vi "Project - Description.vi"(7 "Msg Chain":string, 8 "error in (no error)":errorcluster {"code" format="Error %.0f"}, 10 "Project Doc":refnum<class "Project Documentation.lvclass">, 11 "VIDoc Printer - Confluence In":refnum<class "VIDoc Printer - Confluence.lvclass">) -> (0 "error out":errorcluster {"code" format="Error %.0f"}, 3 "VIDoc Printer - Confluence Out":refnum<class "VIDoc Printer - Confluence.lvclass">)   [LabVIEW 2023, in "VIDoc Printer - Confluence.lvlib" / "VIDoc Printer - Confluence.lvclass"]
uses:
  VIDoc Printer - Confluence.lvclass
  Parsing/Project Documentation/Project Documentation.lvclass
  Confluence Formatting/Types/Format Combo Box.ctl
  Parsing/Project Documentation/Project Documentation.lvclass/Project Documentation.ctl
  Parsing/Project Documentation/Get Description.vi
  VIDoc Printer - Confluence.lvclass/VIDoc Printer - Confluence.ctl
  Confluence Formatting/Confluence Formatting.lvlib
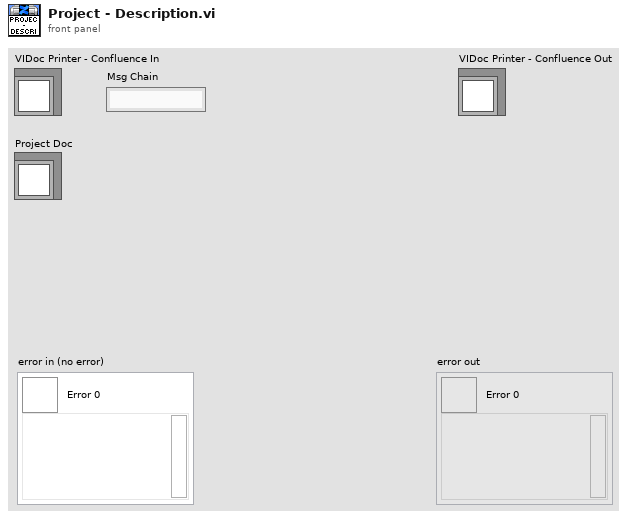
[diagram p1: front panel]
types:
  T1 = typedef "Confluence Formatting.lvlib/Format Combo Box.ctl" = string
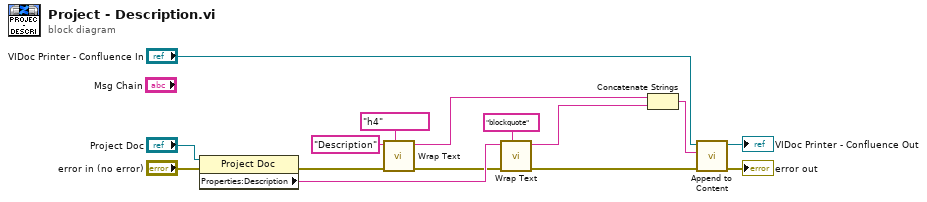
[diagram p0: block diagram]
diagram:
  n1 = property class="Project Doc"(reference="Project Doc", error in="error in (no error)") -> (error out=w11:errorcluster, "Properties:Description"=w13:string)  [unwired: 1 out]
  n2 = call "Wrap Text.vi"("Formatting"=T1 "h4", "Error in"=w11, "String"="Description") -> ("Error out"=w8:errorcluster, "Wrapped String"=w10:string)  [unwired: 7 in]
  n3 = call "Wrap Text.vi"("Formatting"=T1 "blockquote", "Error in"=w8, "String"=w13) -> ("Error out"=w7:errorcluster, "Wrapped String"=w9:string)  [unwired: 7 in]
  n4 = Concatenate Strings(w10, w9) -> (w6:string)
  n5 = call "Append to Content.vi"("error in (no error)"=w7, "Content"=w6, "VIDoc Printer - Confluence In"="VIDoc Printer - Confluence In") -> ("error out"=→"error out":errorcluster, "VIDoc Printer - Confluence Out"=→"VIDoc Printer - Confluence Out":refnum<class "VIDoc Printer - Confluence.lvclass">)  [unwired: 7 in]
